vi "Get Error Message.vi"(11 "Error Interface in":refnum<class "Error Interface.lvclass">) -> (3 "Error Interface out":refnum<class "Error Interface.lvclass">, 4 "Time Stamp":timestamp, 5 "Call Chain":string[](array[string]), 6 "Error Source":string, 7 "Error Message":string)   [LabVIEW 2016, in "Stream Error.lvlib" / "Error Interface.lvclass"]
doc: "--\nCopyright © 2017 Composed SystemsI All rights reserved.\n\nAuthor: Jon McBee <jon.mcbee@composed.io>\n\nThis library is provided \"AS IS\" ,WITHOUT WARRANTIES OR\nCONDITIONS OF ANY KIND, either express or implied.\n\nComposed Systems -- composed.io\n\nStream 0.0.1.1\nJon McBee - Composed Systems\nCopyright (c) 2017, Composed Systems"
uses:
  <userlib>/Composed Systems/Stream/Error/Classes/Error Interface/Error Interface.lvclass
  <userlib>/Composed Systems/Stream/Error/Classes/Error Interface/Error Interface.lvclass/Error Interface.ctl
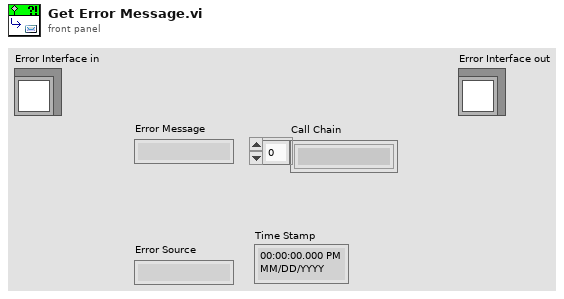
[diagram p1: front panel]
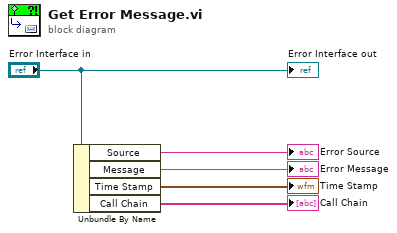
[diagram p0: block diagram]
diagram:
  n1 = Unbundle By Name("Error Interface in") -> ("Source"=→"Error Source":string, "Message"=→"Error Message":string, "Time Stamp"=→"Time Stamp":timestamp, "Call Chain"=→"Call Chain":string[])
  "Error Interface out" <- "Error Interface in"
